vi "Move Labels.vi"(10 "Objects":refnum<vi>[](array[refnum])) -> (2 "Objects dup":refnum<vi>[](array[refnum]))   [LabVIEW 2021, in "_Control To Private Data.lvlib"]
uses:
  _Control To Private Data.lvlib
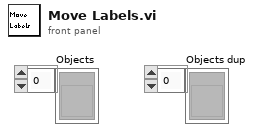
[diagram p1: front panel]
types:
  T1 = typedef "LVRectTypeDef.ctl" = cluster{"Left":i16, "Top":i16, "Right":i16, "Bottom":i16}
  T2 = cluster{"MasterRect":T1, "Label":refnum<vi>, "f":i32, refnum<vi>}
  T3 = enum32{"None", "Size to Fit", "Arrange Horizontally", "Arrange Vertically"}
  T4 = cluster{"Bounds Rect":T1, "Label":refnum<vi>, "f":i32, refnum<vi>}
  T5 = cluster{"Bounds Rect":T1, "Label":refnum<vi>, "right-top":i32, refnum<vi>}
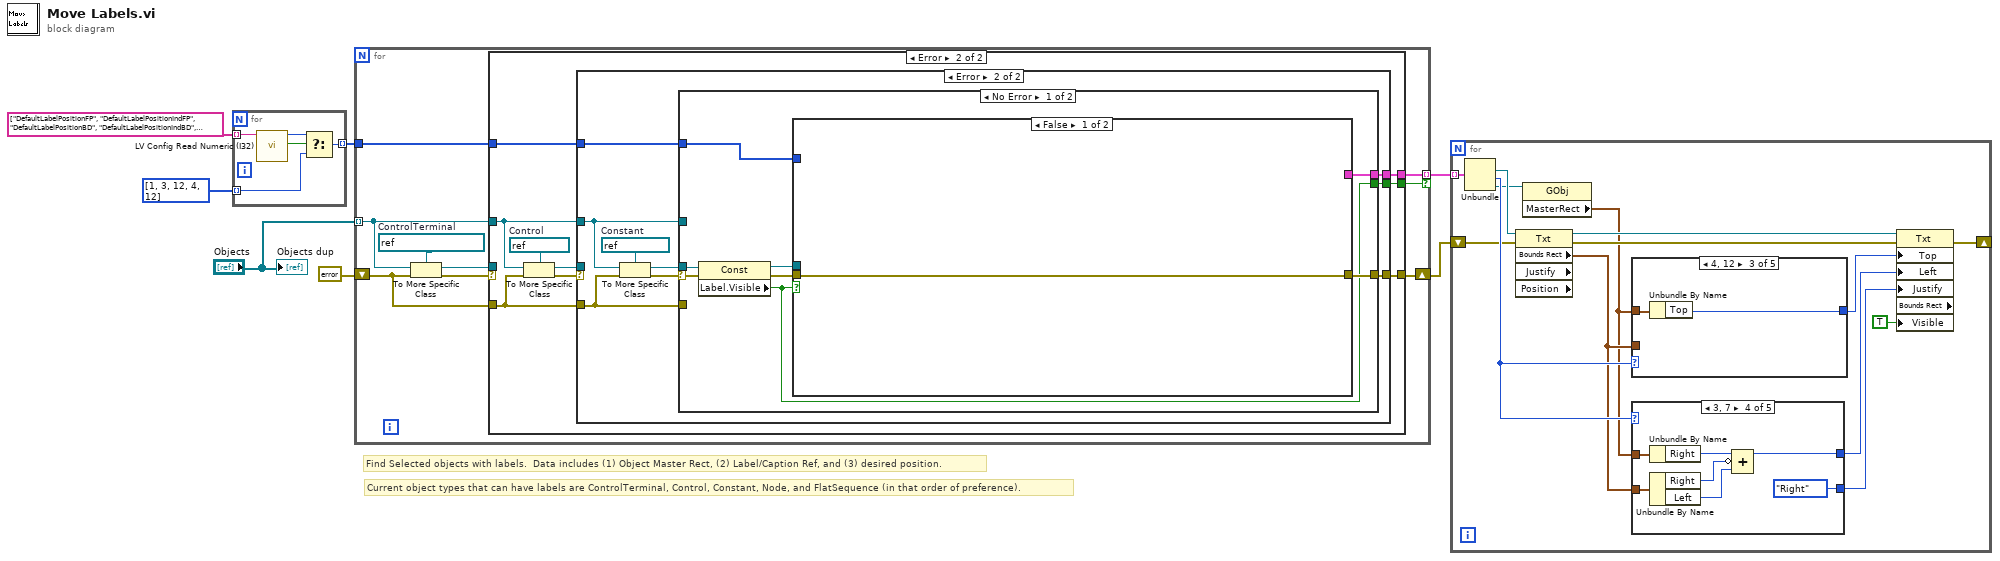
[diagram p0: block diagram]
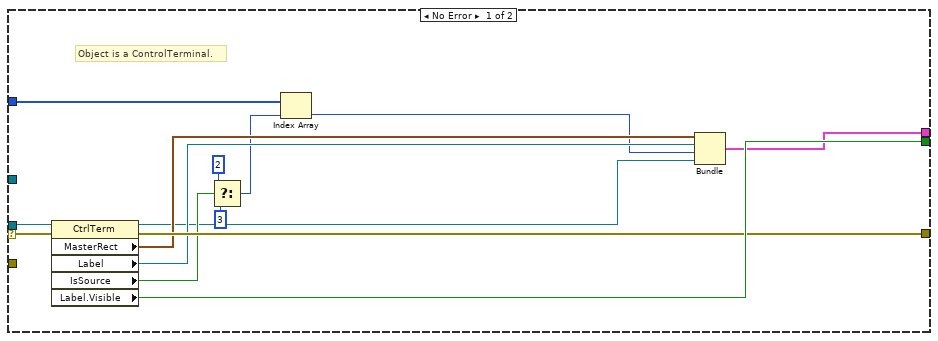
[diagram p2: hidden frame]
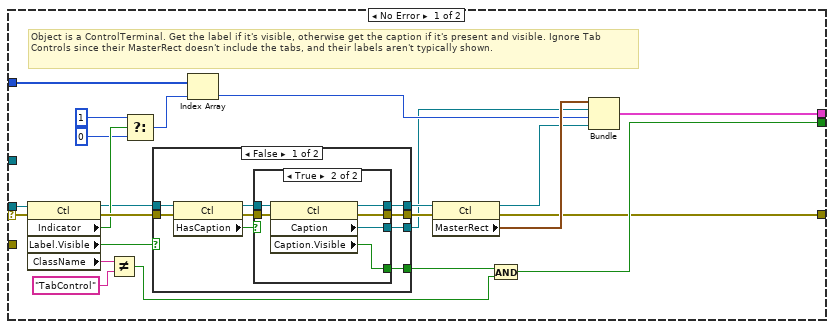
[diagram p3: hidden frame]
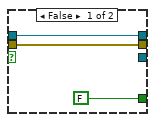
[diagram p4: hidden frame]
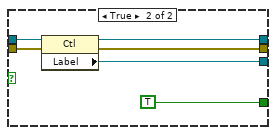
[diagram p5: hidden frame]
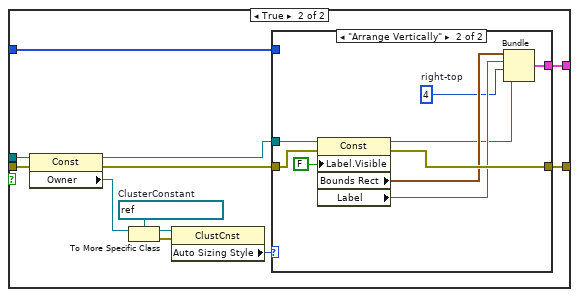
[diagram p6: hidden frame]
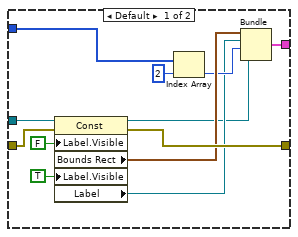
[diagram p7: hidden frame]
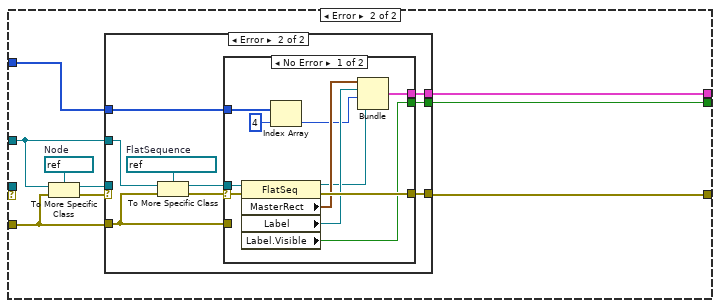
[diagram p8: hidden frame]
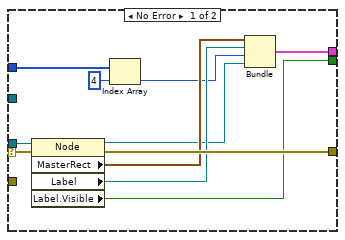
[diagram p9: hidden frame]
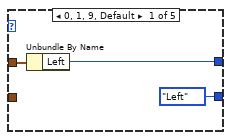
[diagram p11: hidden frame]
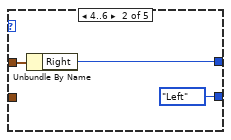
[diagram p12: hidden frame]
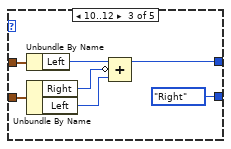
[diagram p13: hidden frame]
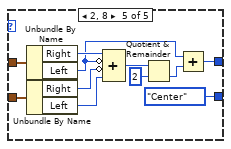
[diagram p14: hidden frame]
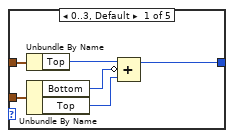
[diagram p15: hidden frame]
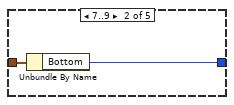
[diagram p16: hidden frame]
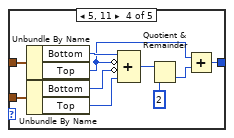
[diagram p17: hidden frame]
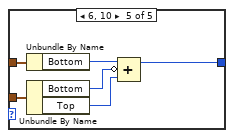
[diagram p18: hidden frame]
diagram:
  # "Current object types that can have labels are ControlTerminal, Control, Constant, Node, and FlatSequence (in that order of preference)."
  # "Find Selected objects with labels.  Data includes (1) Object Master Rect, (2) Label/Caption Ref, and (3) desired position."
  n1 = for {
    tunnel: string[] ["DefaultLabelPositionFP", "DefaultLabelPositionIndFP", "DefaultLabelPositionBD", "DefaultLabelPositionIndBD", "DefaultLabelPositionOtherBD"] -> [w12] mode=indexing
    tunnel: [w9] -> w2 mode=indexing
    tunnel: i32[] [1, 3, 12, 4, 12] -> [w8] mode=indexing
    n2 = call <resource>:"LV Config Read Numeric (I32).vi"("key"=w12) -> ("found?"=w11:bool, "value"=w10:i32)  [unwired: 4 in, 1 out]
    n3 = Select(t=w10, s=w11, f=w8) -> (s? t:f=w9:i32)
  }
  n4 = for {
    shift-right: [w21] -> w3
    shift-left: errorcluster {"status"=FALSE, "code"=0, "source"=""} ("error out") -> [w13]
    tunnel: "Objects" -> [w19] mode=indexing
    tunnel: [w20] -> w6 mode=indexing if=w15
    tunnel: w2 -> [w14]
    w16 = refnum<vi> refnum  # ControlTerminal
    n5 = To More Specific Class(target class=w16, reference=w19, error in=w13) -> (specific class reference=w17:refnum<vi>, error out=w18:errorcluster)
    n6 = case shown="Error" w18 {
      selector: w18 -> [w34 _]
      tunnel: [w32 w41] -> w21
      tunnel: w19 -> [_ w40]
      tunnel: [w29 w39] -> w20
      tunnel: w17 -> [w35 _]
      tunnel: [w33 w37] -> w15
      tunnel: w14 -> [w28 w38]
      tunnel: w13 -> [_ w36]
      frame No Error {
        # "Object is a ControlTerminal."
        n7 = property class="CtrlTerm"(reference=w35, error in=w34) -> (reference out=w22:refnum<vi>, error out=w32:errorcluster, "MasterRect"=w31:T1, "Label"=w30:refnum<vi>, "IsSource"=w27:bool, "Label.Visible"=w33:bool)
        n8 = Select(t=2, s=w27, f=3) -> (s? t:f=w24:i32)
        n9 = Index Array(array=w28, index=w24) -> (element=w23:i32)
        n10 = Bundle("MasterRect"=w31, "Label"=w30, "f"=w23, w22) -> (w29:T2)  [unwired: 1 in]
      }
      frame Error {
        w44 = refnum<vi> refnum  # Control
        n11 = To More Specific Class(target class=w44, reference=w40, error in=w36) -> (specific class reference=w43:refnum<vi>, error out=w42:errorcluster)
        n12 = case shown="Error" w42 {
          selector: w42 -> [w67 _]
          tunnel: w43 -> [w63 _]
          tunnel: [w46 w96] -> w41
          tunnel: w36 -> [_ w97]
          tunnel: w40 -> [_ w95]
          tunnel: [w65 w94] -> w39
          tunnel: w38 -> [w51 w92]
          tunnel: [w48 w93] -> w37
          frame No Error {
            # "Object is a ControlTerminal. Get the label if it's visible, otherwise get the caption if it's present and visible. Ignore Tab Controls since their MasterRect doesn't include the tabs, and their labels aren't typically shown."
            n13 = property class="Ctl"(reference=w63, error in=w67) -> (reference out=w56:refnum<vi>, error out=w64:errorcluster, "Indicator"=w62:bool, "Label.Visible"=w54:bool, "ClassName"=w50:string)
            n14 = Not Equal?(x=w50, y="TabControl") -> (x != y?=w47:bool)
            n15 = Select(t=1, s=w62, f=0) -> (s? t:f=w59:i32)
            n16 = case shown="False" w54 {
              tunnel: w64 -> [w76 w91]
              tunnel: [w73 w88] -> w57
              tunnel: w56 -> [w74 w90]
              tunnel: [w71 w89] -> w55
              tunnel: [w69 w87] -> w53
              tunnel: [w68 TRUE] -> w52
              frame False {
                n17 = property class="Ctl"(reference=w74, error in=w76) -> (reference out=w72:refnum<vi>, error out=w75:errorcluster, "HasCaption"=w70:bool)
                n18 = case shown="True" w70 {
                  tunnel: w75 -> [w78 w85]
                  tunnel: [w78 w84] -> w73
                  tunnel: w72 -> [w79 w83]
                  tunnel: [w79 w82] -> w71
                  tunnel: [_ w81] -> w69
                  tunnel: [FALSE w80] -> w68
                  frame False {
                  }
                  frame True {
                    n19 = property class="Ctl"(reference=w83, error in=w85) -> (reference out=w82:refnum<vi>, error out=w84:errorcluster, "Caption"=w81:refnum<vi>, "Caption.Visible"=w80:bool)
                  }
                }
              }
              frame True {
                n20 = property class="Ctl"(reference=w90, error in=w91) -> (reference out=w89:refnum<vi>, error out=w88:errorcluster, "Label"=w87:refnum<vi>)
              }
            }
            n21 = Index Array(array=w51, index=w59) -> (element=w58:i32)
            n22 = property class="Ctl"(reference=w55, error in=w57) -> (reference out=w45:refnum<vi>, error out=w46:errorcluster, "MasterRect"=w66:T1)
            n23 = And(x=w52, y=w47) -> (x .and. y?=w48:bool)
            n24 = Bundle("MasterRect"=w66, "Label"=w53, "f"=w58, w45) -> (w65:T2)  [unwired: 1 in]
          }
          frame Error {
            w100 = refnum<vi> refnum  # Constant
            n25 = To More Specific Class(target class=w100, reference=w95, error in=w97) -> (specific class reference=w98:refnum<vi>, error out=w99:errorcluster)
            n26 = case shown="No Error" w99 {
              selector: w99 -> [w108 _]
              tunnel: w97 -> [_ w147]
              tunnel: w98 -> [w103 _]
              tunnel: [w107 w148] -> w96
              tunnel: w95 -> [_ w146]
              tunnel: [w106 w145] -> w94
              tunnel: [w101 w144] -> w93
              tunnel: w92 -> [w105 w143]
              frame No Error {
                n27 = property class="Const"(reference=w103, error in=w108) -> (reference out=w102:refnum<vi>, error out=w104:errorcluster, "Label.Visible"=w101:bool)
                n28 = case shown="False" w101 {
                  tunnel: [w109 w121] -> w107
                  tunnel: [_ w120] -> w106
                  tunnel: w105 -> [_ w119]
                  tunnel: w104 -> [w109 w118]
                  tunnel: w102 -> [_ w116]
                  frame False {
                  }
                  frame True {
                    w113 = refnum<vi> refnum  # ClusterConstant
                    n29 = property class="Const"(reference=w116, error in=w118) -> (reference out=w115:refnum<vi>, error out=w117:errorcluster, "Owner"=w114:refnum<vi>)
                    n30 = To More Specific Class(target class=w113, reference=w114) -> (specific class reference=w111:refnum<vi>, error out=w112:errorcluster)  [unwired: 1 in]
                    n31 = property class="ClustCnst"(reference=w111, error in=w112) -> ("Auto Sizing Style"=w110:T3)  [unwired: 2 out]
                    n32 = case shown="\"Arrange Vertically\"" w110 {
                      tunnel: [w133 w142] -> w121
                      tunnel: [w131 w140] -> w120
                      tunnel: w119 -> [w130 _]
                      tunnel: w117 -> [w124 w137]
                      tunnel: w115 -> [w123 w136]
                      frame Default {
                        n33 = property class="Const"(reference=w123, error in=w124, "Label.Visible"=FALSE, "Label.Visible"=TRUE) -> (reference out=w122:refnum<vi>, error out=w133:errorcluster, "Bounds Rect"=w132:T1, "Label"=w127:refnum<vi>)
                        n34 = Index Array(array=w130, index=2) -> (element=w128:i32)
                        n35 = Bundle("Bounds Rect"=w132, "Label"=w127, "f"=w128, w122) -> (w131:T4)  [unwired: 1 in]
                      }
                      frame "Arrange Vertically" {
                        w135 = 4  # right-top
                        n36 = property class="Const"(reference=w136, error in=w137, "Label.Visible"=FALSE) -> (reference out=w134:refnum<vi>, error out=w142:errorcluster, "Bounds Rect"=w141:T1, "Label"=w139:refnum<vi>)
                        n37 = Bundle("Bounds Rect"=w141, "Label"=w139, "right-top"=w135, w134) -> (w140:T5)  [unwired: 1 in]
                      }
                    }
                  }
                }
              }
              frame Error {
                w151 = refnum<vi> refnum  # Node
                n38 = To More Specific Class(target class=w151, reference=w146, error in=w147) -> (specific class reference=w149:refnum<vi>, error out=w150:errorcluster)
                n39 = case shown="Error" w150 {
                  selector: w150 -> [w162 _]
                  tunnel: w149 -> [w160 _]
                  tunnel: [w161 w166] -> w148
                  tunnel: w147 -> [_ w167]
                  tunnel: w146 -> [_ w170]
                  tunnel: [w157 w165] -> w145
                  tunnel: [w156 w163] -> w144
                  tunnel: w143 -> [w155 w164]
                  frame No Error {
                    n40 = property class="Node"(reference=w160, error in=w162) -> (reference out=w152:refnum<vi>, error out=w161:errorcluster, "MasterRect"=w159:T1, "Label"=w158:refnum<vi>, "Label.Visible"=w156:bool)
                    n41 = Index Array(array=w155, index=4) -> (element=w153:i32)
                    n42 = Bundle("MasterRect"=w159, "Label"=w158, "f"=w153, w152) -> (w157:T2)  [unwired: 1 in]
                  }
                  frame Error {
                    w171 = refnum<vi> refnum  # FlatSequence
                    n43 = To More Specific Class(target class=w171, reference=w170, error in=w167) -> (specific class reference=w168:refnum<vi>, error out=w169:errorcluster)
                    n44 = case shown="No Error" w169 {
                      selector: w169 -> [w182 _]
                      tunnel: w168 -> [w181 _]
                      tunnel: w167 -> [_ w183]
                      tunnel: [w180 w183] -> w166
                      tunnel: [w177 _] -> w165
                      tunnel: w164 -> [w176 _]
                      tunnel: [w173 _] -> w163
                      frame No Error {
                        n45 = property class="FlatSeq"(reference=w181, error in=w182) -> (reference out=w172:refnum<vi>, error out=w180:errorcluster, "MasterRect"=w179:T1, "Label"=w178:refnum<vi>, "Label.Visible"=w173:bool)
                        n46 = Index Array(array=w176, index=4) -> (element=w174:i32)
                        n47 = Bundle("MasterRect"=w179, "Label"=w178, "f"=w174, w172) -> (w177:T2)  [unwired: 1 in]
                      }
                      frame Error {
                      }
                    }
                  }
                }
              }
            }
          }
        }
      }
    }
  }
  n48 = for {
    tunnel: w6 -> [w197] mode=indexing
    shift-right: [w184] -> _
    shift-left: w3 -> [w194]
    n49 = Unbundle(w197) -> ("Label"=w195:refnum<vi>, "f"=w196:i32, w185:refnum<vi>)  [unwired: 1 out]
    n50 = property class="Txt" props=["Bounds Rect", "Justify", "Position"](reference=w195, error in=w194) -> (reference out=w193:refnum<vi>, error out=w191:errorcluster, "Bounds Rect"=w190:T1)  [unwired: 2 out]
    n51 = property class="GObj"(reference=w185) -> ("MasterRect"=w186:T1)  [unwired: 1 in, 2 out]
    n52 = case shown="4, 12" w196 {
      tunnel: w186 -> [w234 w236 w238 w248 w254]
      tunnel: w190 -> [w233 _ _ w247 w253]
      tunnel: [w229 w235 w237 w243 w249] -> w192
      frame 0..3, Default {
        n53 = Unbundle By Name(w234) -> ("Top"=w232:i16)
        n54 = Unbundle By Name(w233) -> ("Bottom"=w231:i16, "Top"=w230:i16)
        n55 = Compound Arithmetic op=ADD(w232, invert w231, w230) -> (w229:i16)
      }
      frame 7..9 {
        n56 = Unbundle By Name(w236) -> ("Bottom"=w235:i16)
      }
      frame 4, 12 {
        n57 = Unbundle By Name(w238) -> ("Top"=w237:i16)
      }
      frame 5, 11 {
        n58 = Unbundle By Name(w248) -> ("Bottom"=w242:i16, "Top"=w241:i16)
        n59 = Unbundle By Name(w247) -> ("Bottom"=w246:i16, "Top"=w245:i16)
        n60 = Compound Arithmetic op=ADD(w242, invert w241, invert w246, w245) -> (w240:i16)
        n61 = Quotient & Remainder(x=w240, y=i16 2) -> (floor(x/y)=w244:i16)  [unwired: 1 out]
        n62 = Add(x=w241, y=w244) -> (x+y=w243:i16)
      }
      frame 6, 10 {
        n63 = Unbundle By Name(w254) -> ("Bottom"=w252:i16)
        n64 = Unbundle By Name(w253) -> ("Bottom"=w251:i16, "Top"=w250:i16)
        n65 = Compound Arithmetic op=ADD(w252, invert w251, w250) -> (w249:i16)
      }
    }
    n66 = case shown="3, 7" w196 {
      tunnel: w186 -> [w200 w203 w210 w217 w226]
      tunnel: w190 -> [_ _ w208 w215 w225]
      tunnel: [w199 w202 w205 w212 w222] -> w189
      tunnel: [enum16{"Left", "Center", "Right"}."Left" ("Justification") enum16{"Left", "Center", "Right"}."Left" ("Justification") enum16{"Left", "Center", "Right"}."Right" ("Justification") enum16{"Left", "Center", "Right"}."Right" ("Justification") enum16{"Left", "Center", "Right"}."Center" ("Justification")] -> w188
      frame 0, 1, 9, Default {
        n67 = Unbundle By Name(w200) -> ("Left"=w199:i16)
      }
      frame 4..6 {
        n68 = Unbundle By Name(w203) -> ("Right"=w202:i16)
      }
      frame 10..12 {
        n69 = Unbundle By Name(w210) -> ("Left"=w209:i16)
        n70 = Unbundle By Name(w208) -> ("Right"=w207:i16, "Left"=w206:i16)
        n71 = Compound Arithmetic op=ADD(w209, invert w207, w206) -> (w205:i16)
      }
      frame 3, 7 {
        n72 = Unbundle By Name(w217) -> ("Right"=w216:i16)
        n73 = Unbundle By Name(w215) -> ("Right"=w214:i16, "Left"=w213:i16)
        n74 = Compound Arithmetic op=ADD(w216, invert w214, w213) -> (w212:i16)
      }
      frame 2, 8 {
        n75 = Unbundle By Name(w226) -> ("Right"=w224:i16, "Left"=w221:i16)
        n76 = Unbundle By Name(w225) -> ("Right"=w227:i16, "Left"=w228:i16)
        n77 = Compound Arithmetic op=ADD(w224, invert w221, invert w227, w228) -> (w219:i16)
        n78 = Quotient & Remainder(x=w219, y=i16 2) -> (floor(x/y)=w223:i16)  [unwired: 1 out]
        n79 = Add(x=w221, y=w223) -> (x+y=w222:i16)
      }
    }
    n80 = property class="Txt" props=["Top", "Left", "Justify", "Bounds Rect", "Visible"](reference=w193, error in=w191, "Top"=w192, "Left"=w189, "Justify"=w188, "Visible"=TRUE) -> (error out=w184:errorcluster)  [unwired: 2 out]
  }
  "Objects dup" <- "Objects"
